vi "SearchForAllTests (In Memory).vi"() -> ()   [LabVIEW 2013, in "Caraya.lvlib" / "Test Runner.lvclass"]
uses:
  classes/Test Runner/Test Runner.lvclass
  classes/Test/Define Test.vi
  classes/Test/Test.lvclass
panel:
  out "Top Level Tests":string[](array[string])
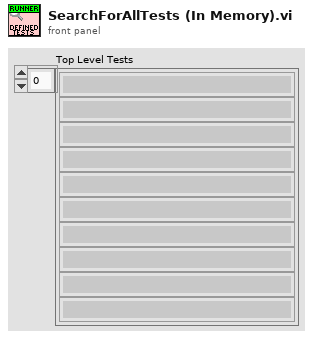
[diagram p1: front panel]
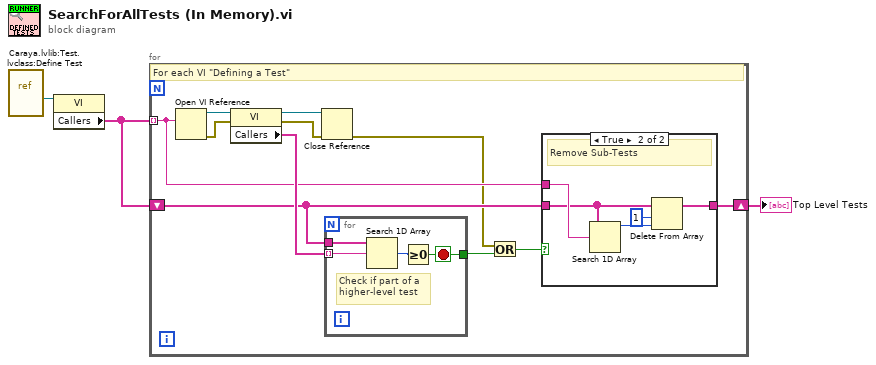
[diagram p0: block diagram]
diagram:
  n1 = vi-ref "Caraya.lvlib:Test.lvclass:Define Test.vi"() -> (w3:refnum<vi>)
  n2 = property class="VI"(reference=w3) -> ("Callers"=w2:string[])  [unwired: 1 in, 2 out]
  n3 = for {
    shift-right: [w8] -> w1
    shift-left: w2 -> [w9]
    tunnel: w2 -> [w7] mode=indexing
    # "For each VI \"Defining a Test\""
    n4 = Open VI Reference(vi path=w7) -> (vi reference=w14:refnum<vi>, error out=w11:errorcluster)  [unwired: 5 in]
    n5 = property class="VI"(reference=w14, error in=w11) -> (reference out=w13:refnum<vi>, error out=w10:errorcluster, "Callers"=w12:string[])
    n6 = Close Reference(reference=w13, error in (no error)=w10) -> (error out=w6:errorcluster)
    n7 = for {
      tunnel: w9 -> [w24]
      tunnel: w12 -> [w23] mode=indexing
      tunnel: [w21] -> w4
      stop <- w21 stop-if-true
      # "Check if part of a\nhigher-level test"
      n8 = Search 1D Array(1D array=w24, element=w23) -> (index of element=w22:i32)  [unwired: 1 in]
      n9 = Greater Or Equal To 0?(x=w22) -> (x >= 0?=w21:bool)
    }
    n10 = Or(x=w6, y=w4) -> (x .or. y?=w5:bool)
    n11 = case shown="True" w5 {
      tunnel: w9 -> [w15 w19]
      tunnel: [w15 w16] -> w8
      tunnel: w7 -> [_ w20]
      frame False {
      }
      frame True {
        # "Remove Sub-Tests"
        n12 = Search 1D Array(1D array=w19, element=w20) -> (index of element=w18:i32)  [unwired: 1 in]
        n13 = Delete From Array(array=w19, length=1, index=w18) -> (array with subset deleted=w16:string[])  [unwired: 1 out]
      }
    }
  }
  "Top Level Tests" <- w1
